vi "LED_WRITE.vi"(0 "I2C Ref":string="My I2C RefNum", 1 "I2CRegister":u8, 2 "Alliance":enum16{"Red", "Blue"}(ring), 3 "Robot Mode":T1(ring), 4 "Lift Position":u8=35) -> (5 "I2C Byte Output Array":u8[](array[numeric]), 6 "error out":errorcluster)   [LabVIEW 2013]
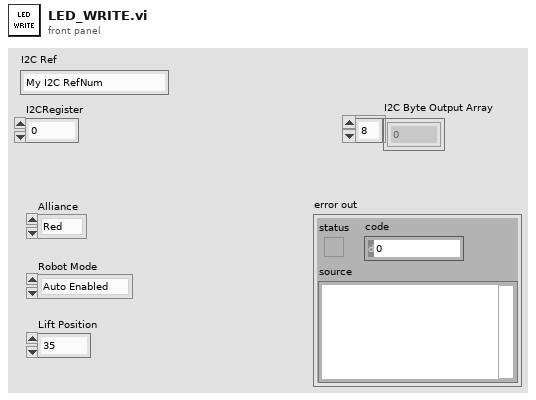
[diagram p1: front panel]
types:
  T1 = enum16{"Auto Enabled", "Auto Disabled", "Teleop Enabled", "Teleop Disabled", "Test Enabled", "Test Disabled", "Disconnected", "Error", "Finished"}
  T2 = typedef "WPI_I2CDevRef.ctl" = cluster{"DevStatus":errorcluster, "Digital Module":T3, "Device Address":u8}
  T3 = typedef "FPGA_TypedefDigitalModule.ctl" = enum16{"Digital Module 1", "Digital Module 2"}
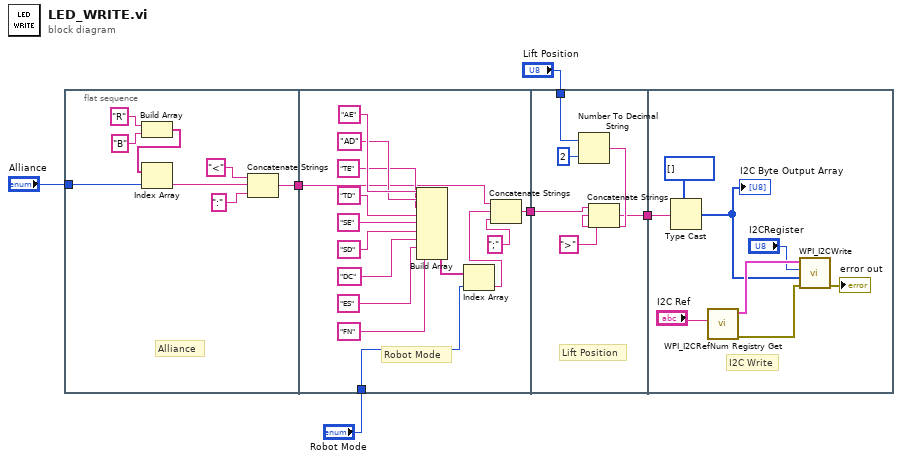
[diagram p0: block diagram]
diagram:
  n1 = flat-sequence {
    tunnel: "Alliance" -> [w12]
    tunnel: [w7] -> w5
    tunnel: w5 -> [w17]
    tunnel: [w16] -> w3
    tunnel: "Robot Mode" -> [w15]
    tunnel: "Lift Position" -> [w35]
    tunnel: w3 -> [w33]
    tunnel: [w30] -> w2
    tunnel: w2 -> [w42]
    frame #0 {
      # "Alliance"
      n2 = Build Array("R", "B") -> (w11:string[])
      n3 = Index Array(array=w11, index=w12) -> (element=w9:string)
      n4 = Concatenate Strings("<", w9, ":") -> (w7:string)
    }
    frame #1 {
      # "Robot Mode"
      n5 = Build Array("AE", "AD", "TE", "TD", "SE", "SD", "DC", "ES", "FN") -> (w20:string[])
      n6 = Index Array(array=w20, index=w15) -> (element=w18:string)
      n7 = Concatenate Strings(w17, w18, ";" ("element")) -> (w16:string)
    }
    frame #2 {
      # "Lift Position"
      n8 = Number To Decimal String(number=w35, width (-)=i16 2) -> (decimal integer string=w32:string)
      n9 = Concatenate Strings(w33, w32, ">") -> (w30:string)
    }
    frame #3 {
      # "I2C Write"
      n10 = Type Cast(type=u8[] [], x=w42) -> (*(type *) &x=w39:u8[])
      "I2C Byte Output Array" <- w39
      n11 = call <vilib>:"WPI_I2CRefNum Registry Get.vi"("refnum name"="I2C Ref") -> ("error out"=w37:errorcluster, "I2CDevRef"=w40:T2)  [unwired: 9 in]
      n12 = call <vilib>:"WPI_I2CWrite.vi"("error in (no error)"=w37, "I2CDataToSend"=w39, "I2CRegister"="I2CRegister", "I2CDevRef"=w40) -> ("error out"=→"error out":errorcluster)  [unwired: 6 in, 1 out]
    }
  }
